vi "CurrentAv+Charge(SubVI).vi"(6 "old current value":dbl, 9 "old charge value":dbl, 10 "new current value":dbl, 11 "cycle time":dbl) -> (2 "charge":dbl, 3 "current average":dbl)   [LabVIEW 2017]
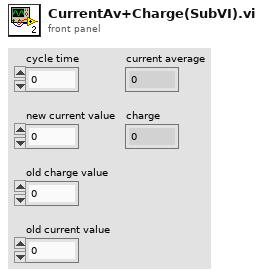
[diagram p1: front panel]
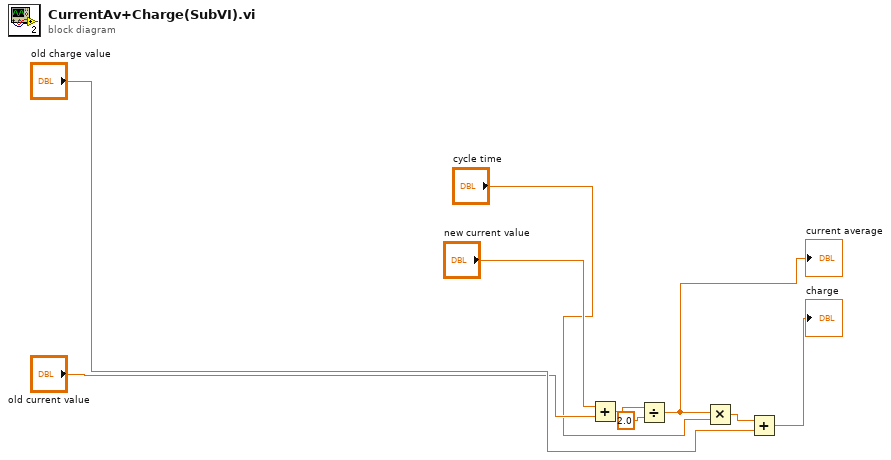
[diagram p0: block diagram]
diagram:
  n1 = Add(x="new current value", y="old current value") -> (x+y=w1:dbl)
  n2 = Divide(x=w1, y=2.0) -> (x/y=w9:dbl)
  "current average" <- w9
  n3 = Multiply(x=w9, y="cycle time") -> (x*y=w6:dbl)
  n4 = Add(x=w6, y="old charge value") -> (x+y=→"charge":dbl)
